vi "Slice Engine.vi"(7 "System Parameters":T1={"Optical Parameters"={"Obj. Focal Length [mm]"=0.0, "Scan Lens EFL[mm]"=0.0, "Tube Lens EFL[mm]"=0.0, "Galvo V Range (+/-)"=0.0, "Galvo Max Half Angle [Deg]"=0.0, "Max Galvo Range[%]"=0.0}, "Vibratome"={"Z Bottom [mm]"=0.0, "Pre Cut Dwell [s]"=0.0, "Blade Frequency [RPM]"=0, "Slice Speed [mm/s]"=0.0, "Post Cut Dwell [s]"=0.0, "Ramp Time [s]"=0.0, "Start X [mm]"=0.0, "Start Y [mm]"=0.0, "Slice Length [mm]"=0.0, "Slice Axis"=enum."X Axis", "Controller VISA Ref"="COM4"}, "Table Stages"={"X Stage"={"Position"=0.0, "Is.Enabled?"=FALSE, "Is.Connected?"=FALSE, "Device SN"="45876425", "AccelerationMaximum"=50.0, "VelocityMaximum"=50.0, "Acceleration"=50.0, "Velocity"=50.0, "waitTimeout (ms)"=500000, "Model"=enum."Thorlabs LTS", "Is.Homed?"=FALSE}, "Y Stage"={"Position"=0.0, "Is.Enabled?"=FALSE, "Is.Connected?"=FALSE, "Device SN"="45995820", "AccelerationMaximum"=50.0, "VelocityMaximum"=50.0, "Acceleration"=50.0, "Velocity"=50.0, "waitTimeout (ms)"=500000, "Model"=enum."Thorlabs LTS", "Is.Homed?"=FALSE}, "Z Stage"={"Position"=0.0, "Is.Enabled?"=FALSE, "Is.Connected?"=FALSE, "Device SN"="49103464", "AccelerationMaximum"=10.0, "VelocityMaximum"=5.0, "Acceleration"=10.0, "Velocity"=5.0, "waitTimeout (ms)"=100000, "Model"=enum."Thorlabs MLJ", "Is.Homed?"=FALSE}}, "Imaging Parameter"={"Raster Scan Direction"=enum."Uni Directional", "Pixel Dwell Time [Clock Cycles]"=0, "Flyback Time [Clock Cycles]"=0, "XY Center [um]"={"X"=1.0, "Y"=1.0}, "Pixel Step Size [um]"=0.0, "XY Image Size"=enum."32 x 32", "Custom"=FALSE, "Custom Size"={"X"=1, "Y"=1}, "Line Averages"=1}, "Galvo HW Parameters"={"Analog Out Channel"="GalvoCtrl/ao0,GalvoCtrl/ao1", "Min Voltage"=-10.0, "Max Voltage"=10.0, "Pixel Clock Source"="/GalvoCtrl/PFI0", "Sample Rate"=1000.0, "Line Clock Out Ch"="GalvoCtrl/port0/line0"}, "Alazar parameters"={"Trigger Settings"={"General Trigger Settings"={"Trigger Operation"=0, "Coupling ID"=2, "Range ID"=2, "Delay"=0, "Timeout Ticks"=0, "Mode"=1, "Parameter"=1}, "Trigger Engine 1"={"Trigger Engine"=0, "Source"=2, "Slope"=1, "Level"=140}, "Trigger Engine 2"={"Trigger Engine"=1000, "Source"=2048, "Slope"=2048, "Level"=140}}, "Capture Clock"={"Sample Rate"=100, "Decimation"=0, "Source"=2, "Edge"=0}, "Device ID"={"System ID"=1, "Board ID"=1}, "Ch A Input Control"={"Channel"=1, "Coupling"=2, "Range"=10, "Impedance"=2}, "Ch B Input Control"={"Channel"=2, "Coupling"=2, "Range"=10, "Impedance"=2}, "Acq Settings"={"Window Type"=1, "Record Length"=1440, "Footer"=0, "Offset"=0, "Records Per Buffer"=2048, "Samples per record"=2048, "Records Count (Records/Acq)"=2147483647, "Output Format"=10}}, "Mosaic Paramter"={"X Axis"={"Start [mm]"=0.0, "Steps [pts]"=0.0, "End [mm]"=0.0}, "Y Axis"={"Start [mm]"=0.0, "Steps [pts]"=0.0, "End [mm]"=0.0}, "Scan Pattern"=enum."Uni-directional", "Overlap Options"={"Overlap Type"=enum."No Overlap", "Percent Overlap"=0, "Justify"=enum."Start"}}, "Vibratome Axis"={"Start [mm]"=95.8, "thick[um]"=2.1, "#slices"=111}} {"Alazar parameters"."Acq Settings"."Output Format" items=["U16_LOG"=1, "U16_AMP2"=257]; "Alazar parameters"."Acq Settings"."Window Type" items=["DSP_WINDOW_NONE", "DSP_WINDOW_HANNING", "DSP_WINDOW_HAMMING", "DSP_WINDOW_BLACKMAN", "DSP_WINDOW_BLACKMAN_HARRIS", "DSP_WINDOW_BARTLETT"]; "Alazar parameters"."Acq Settings"."Footer" items=["FOOTER_NONE", "FOOTER_NPT"]; "Alazar parameters"."Ch B Input Control"."Channel" items=["A"=1, "B"=2, "C"=4, "D"=8]; "Alazar parameters"."Ch B Input Control"."Coupling" items=["AC"=1, "DC"=2]; "Alazar parameters"."Ch B Input Control"."Range" items=["20 mV"=1, "40 mV"=2, "50 mV"=3, "80 mV"=4, "100 mV"=5, "200 mV"=6, "400 mV"=7, "500 mV"=8, "800 mV"=9, "1 V"=10, "1.25 V"=33, "2 V"=11, "4 V"=12, "5 V"=13, "8 V"=14, "10 V"=15, "20 V"=16]; "Alazar parameters"."Ch B Input Control"."Impedance" items=["1 MOhm"=1, "50 Ohm"=2, ""=0]; "Alazar parameters"."Ch A Input Control"."Channel" items=["A"=1, "B"=2, "C"=4, "D"=8]; "Alazar parameters"."Ch A Input Control"."Coupling" items=["AC"=1, "DC"=2]; "Alazar parameters"."Ch A Input Control"."Range" items=["20 mV"=1, "40 mV"=2, "50 mV"=3, "80 mV"=4, "100 mV"=5, "200 mV"=6, "400 mV"=7, "500 mV"=8, "800 mV"=9, "1 V"=10, "1.25 V"=33, "2 V"=11, "4 V"=12, "5 V"=13, "8 V"=14, "10 V"=15, "20 V"=16]; "Alazar parameters"."Ch A Input Control"."Impedance" items=["1 MOhm"=1, "50 Ohm"=2, ""=0]; "Alazar parameters"."Capture Clock"."Edge" items=["Rising", "Falling"]; "Alazar parameters"."Capture Clock"."Source" items=["Internal"=1, "Fast External"=2, "Medium External"=3, "Slow External"=4, "External AC"=5, "External DC"=6, "External 10MHz"=7]; "Alazar parameters"."Trigger Settings"."General Trigger Settings"."Trigger Operation" items=["J", "K", "J OR K", "J AND K", "J XOR K", "J AND NOT K", "NOT J AND K"]; "Alazar parameters"."Trigger Settings"."General Trigger Settings"."Coupling ID" items=["AC"=1, "DC"=2]; "Alazar parameters"."Trigger Settings"."General Trigger Settings"."Range ID" items=["5 V", "1 V", "TTL"]; "Alazar parameters"."Trigger Settings"."Trigger Engine 1"."Trigger Engine" items=["J", "K"]; "Alazar parameters"."Trigger Settings"."Trigger Engine 1"."Source" items=["A", "B", "External", "Disable", "C", "D"]; "Alazar parameters"."Trigger Settings"."Trigger Engine 1"."Slope" items=["Positive"=1, "Negative"=2]; "Alazar parameters"."Trigger Settings"."Trigger Engine 2"."Trigger Engine" items=["J", "K"]; "Alazar parameters"."Trigger Settings"."Trigger Engine 2"."Source" items=["A", "B", "External", "Disable", "C", "D"]; "Alazar parameters"."Trigger Settings"."Trigger Engine 2"."Slope" items=["Positive"=1, "Negative"=2]; "Imaging Parameter"."Line Averages" min=1 max=30 step=1; "Imaging Parameter"."Flyback Time [Clock Cycles]" max=10 step=1; "Imaging Parameter"."Pixel Step Size [um]" min=0.0 max=10.0 step=0.01; "Imaging Parameter"."Custom Size"."Y" min=1 max=30 step=1; "Imaging Parameter"."Custom Size"."X" min=1 max=30 step=1; "Imaging Parameter"."XY Center [um]"."Y" min=1.0 max=30.0 step=1.0; "Imaging Parameter"."XY Center [um]"."X" min=1.0 max=30.0 step=1.0; "Imaging Parameter"."Pixel Dwell Time [Clock Cycles]" max=10 step=1}, 8 "error in (no error)":errorcluster, 11 "Last Slice?":bool) -> (0 "error out":errorcluster)   [LabVIEW 2018]
uses:
  Controls/System Parameters.ctl
  Controls/Optical Parameters.ctl
  Controls/Vibratome Parameters.ctl
  Controls/Translation Stage Parameters.ctl
  Hardware Mfg/Thorlabs Translation Stages/Controls/Translation Stage Cluster.ctl
  Controls/Translation Stage Types.ctl
  Controls/Imaging Parameters.ctl
  Controls/Scan Direction.ctl
  type defines/Alazar parameters.ctl
  Hardware Mfg/AlazarTech SDK/Controls/General Trigger Settings.ctl
  Hardware Mfg/AlazarTech SDK/Controls/Trigger Engine Controls.ctl
  Hardware Mfg/AlazarTech SDK/Controls/Clock Controls.ctl
  Hardware Mfg/AlazarTech SDK/Controls/Alazar Device ID.ctl
  Hardware Mfg/AlazarTech SDK/Controls/Channel Input Controls.ctl
  Hardware Mfg/AlazarTech SDK/Controls/Alazar Acquisition Settings.ctl
  Controls/Queue Manager Actions.ctl
  Controls/QueueNames.ctl
  Hardware Mfg/Thorlabs Translation Stages/Controls/Motion Translation Module Control.ctl
  Controls/Set Get Controls.ctl
panel:
  # "X"
  # "X"
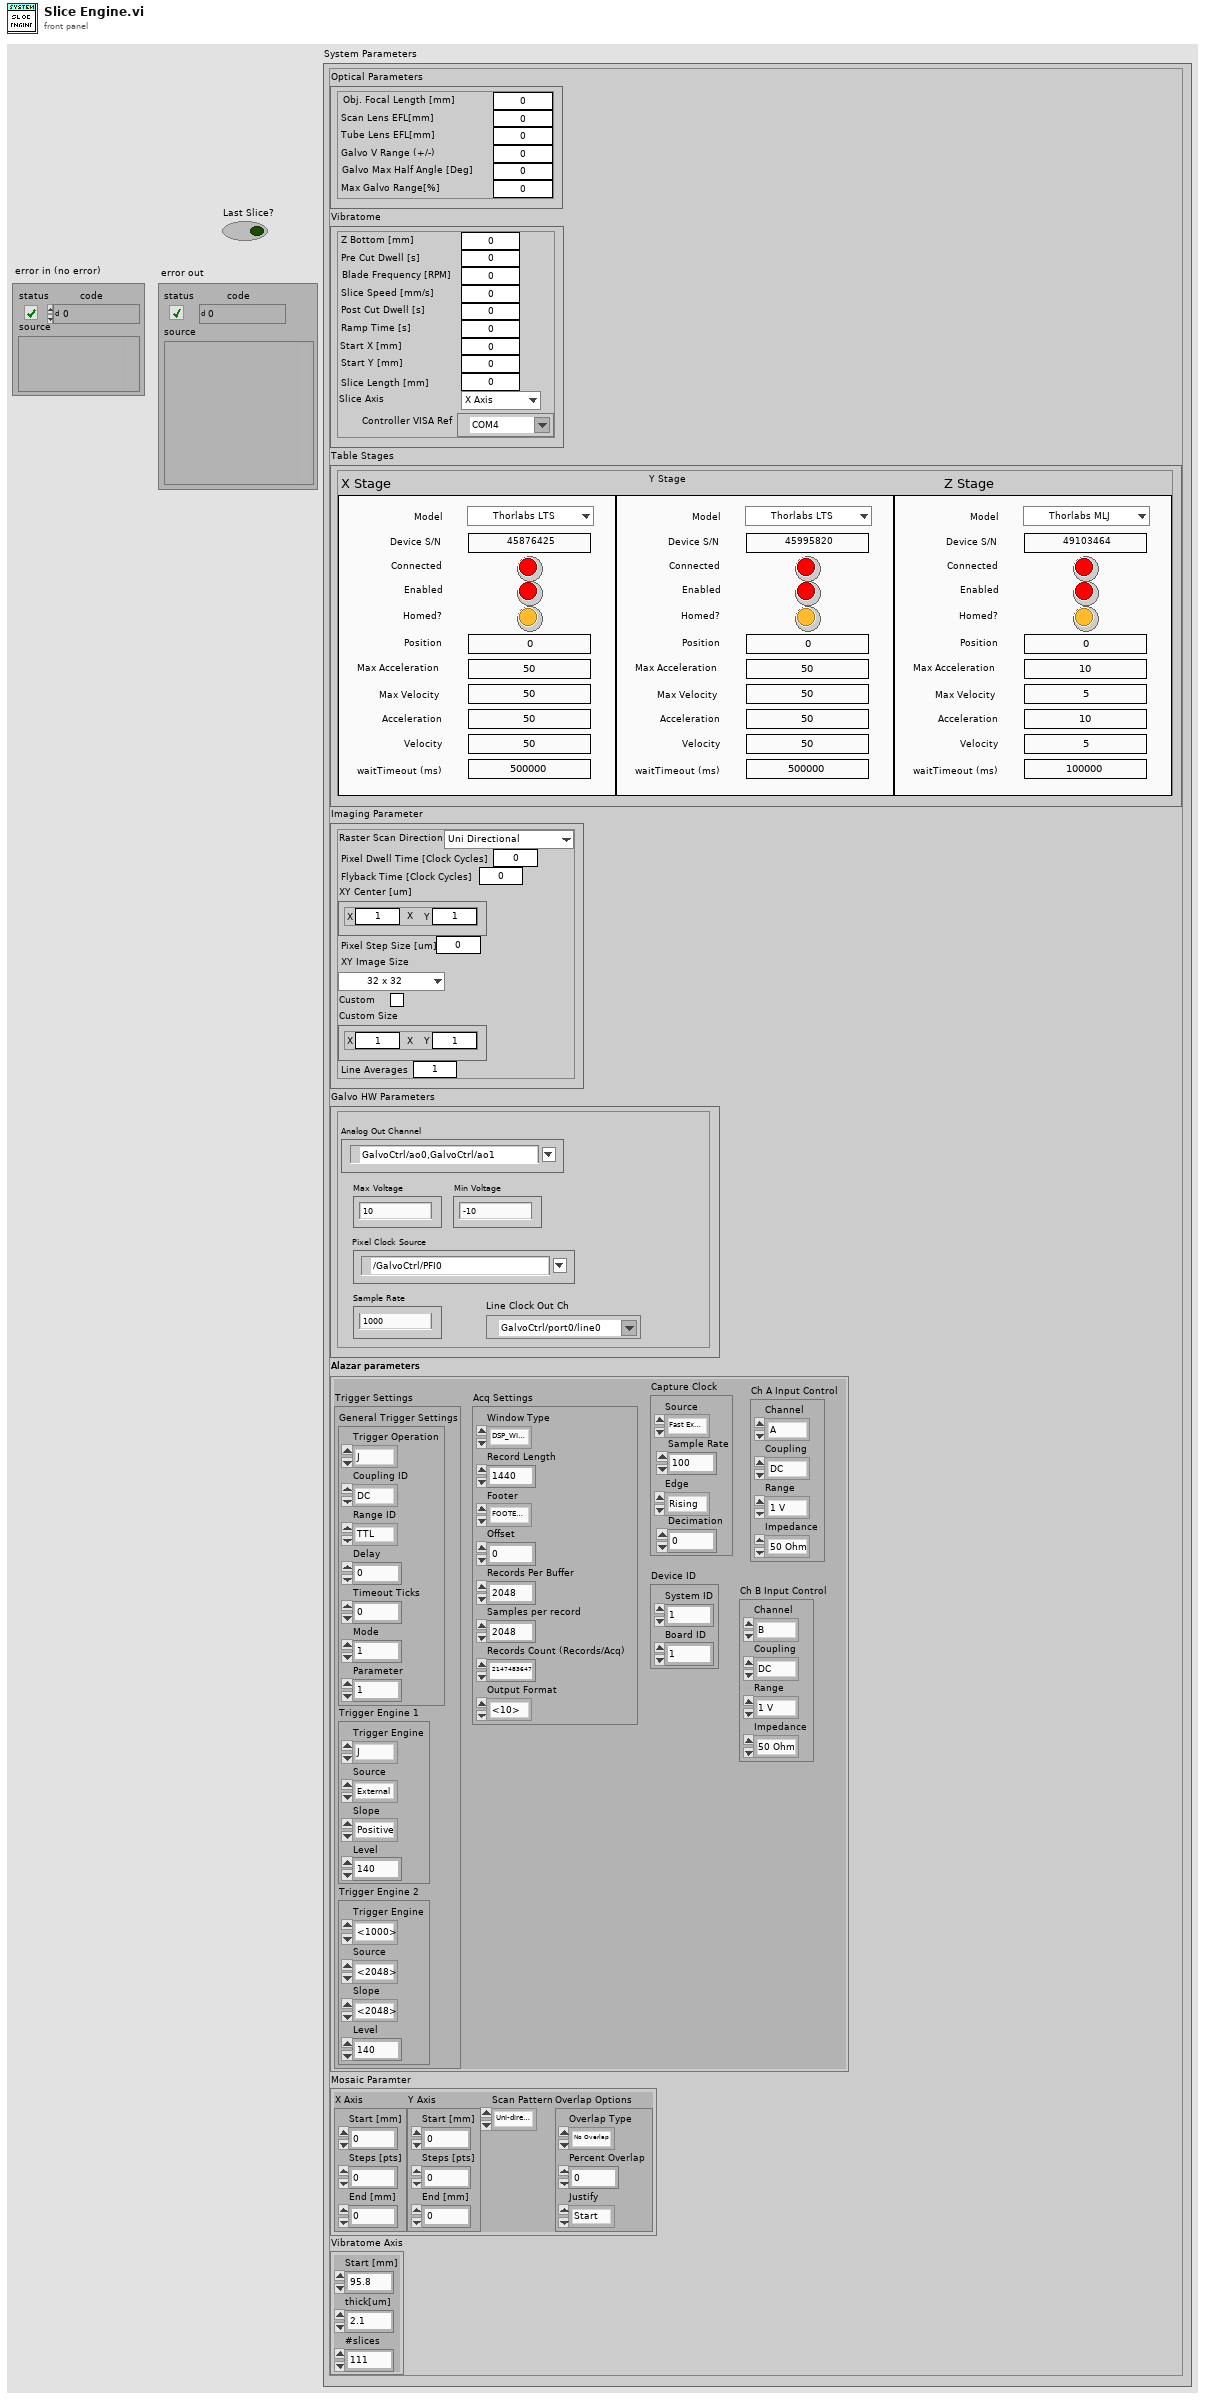
[diagram p1: front panel]
types:
  T1 = typedef "System Parameters.ctl" = cluster{"Optical Parameters":T2, "Vibratome":T3, "Table Stages":T4, "Imaging Parameter":T7, "Galvo HW Parameters":cluster{"Analog Out Channel":tag, "Min Voltage":dbl, "Max Voltage":dbl, "Pixel Clock Source":tag, "Sample Rate":dbl, "Line Clock Out Ch":tag}, "Alazar parameters":T9, "Mosaic Paramter":cluster{"X Axis":cluster{"Start [mm]":dbl, "Steps [pts]":dbl, "End [mm]":dbl}, "Y Axis":cluster{"Start [mm]":dbl, "Steps [pts]":dbl, "End [mm]":dbl}, "Scan Pattern":enum16{"Uni-directional", "Bi-Directional", "Spiral Out", "Spiral In"}, "Overlap Options":cluster{"Overlap Type":enum16{"No Overlap", "X Only", "Y Only", "X and Y"}, "Percent Overlap":u8, "Justify":enum16{"Start", "Center", "End"}}}, "Vibratome Axis":cluster{"Start [mm]":dbl, "thick[um]":dbl, "#slices":u16}}
  T2 = typedef "Optical Parameters.ctl" = cluster{"Obj. Focal Length [mm]":dbl, "Scan Lens EFL[mm]":dbl, "Tube Lens EFL[mm]":dbl, "Galvo V Range (+/-)":dbl, "Galvo Max Half Angle [Deg]":dbl, "Max Galvo Range[%]":dbl}
  T3 = typedef "Vibratome Parameters.ctl" = cluster{"Z Bottom [mm]":dbl, "Pre Cut Dwell [s]":dbl, "Blade Frequency [RPM]":u16, "Slice Speed [mm/s]":dbl, "Post Cut Dwell [s]":dbl, "Ramp Time [s]":dbl, "Start X [mm]":dbl, "Start Y [mm]":dbl, "Slice Length [mm]":dbl, "Slice Axis":enum16{"X Axis", "Y Axis", "Z Axis"}, "Controller VISA Ref":refnum<visa-resource-name>}
  T4 = typedef "Translation Stage Parameters.ctl" = cluster{"X Stage":T5, "Y Stage":T5, "Z Stage":T5}
  T5 = typedef "Translation Stage Cluster.ctl" = cluster{"Position":dbl, "Is.Enabled?":bool, "Is.Connected?":bool, "Device SN":string, "AccelerationMaximum":dbl, "VelocityMaximum":dbl, "Acceleration":dbl, "Velocity":dbl, "waitTimeout (ms)":i32, "Model":T6, "Is.Homed?":bool}
  T6 = typedef "Translation Stage Types.ctl" = enum16{"None", "Thorlabs LTS", "Thorlabs MLJ"}
  T7 = typedef "Imaging Parameters.ctl" = cluster{"Raster Scan Direction":T8, "Pixel Dwell Time [Clock Cycles]":u16, "Flyback Time [Clock Cycles]":u16, "XY Center [um]":cluster{"X":dbl, "Y":dbl}, "Pixel Step Size [um]":dbl, "XY Image Size":enum16{"32 x 32", "64 x 64", "128 x 128", "256 x 256", "512 x 512", "1024 x 1024", "2048 x 2048"}, "Custom":bool, "Custom Size":cluster{"X":u16, "Y":u16}, "Line Averages":u8}
  T8 = typedef "Scan Direction.ctl" = enum16{"Uni Directional", "Bi Directional", "None"}
  T9 = typedef "Alazar parameters.ctl" = cluster{"Trigger Settings":cluster{"General Trigger Settings":T10, "Trigger Engine 1":T11, "Trigger Engine 2":T11}, "Capture Clock":T12, "Device ID":T13, "Ch A Input Control":T14, "Ch B Input Control":T14, "Acq Settings":T15}
  T10 = typedef "General Trigger Settings.ctl" = cluster{"Trigger Operation":u32, "Coupling ID":u32, "Range ID":u32, "Delay":u32, "Timeout Ticks":u32, "Mode":u32, "Parameter":u32}
  T11 = typedef "Trigger Engine Controls.ctl" = cluster{"Trigger Engine":u32, "Source":u32, "Slope":u32, "Level":u32}
  T12 = typedef "Clock Controls.ctl" = cluster{"Sample Rate":u32, "Decimation":u32, "Source":u32, "Edge":u32}
  T13 = typedef "Alazar Device ID.ctl" = cluster{"System ID":u32, "Board ID":u32}
  T14 = typedef "Channel Input Controls.ctl" = cluster{"Channel":u8, "Coupling":u32, "Range":u32, "Impedance":u32}
  T15 = typedef "Alazar Acquisition Settings.ctl" = cluster{"Window Type":u32, "Record Length":u32, "Footer":u32, "Offset":u32, "Records Per Buffer":u32, "Samples per record":u32, "Records Count (Records/Acq)":u32, "Output Format":u32}
  T16 = typedef "QueueNames.ctl" = enum16{"Main GUI", "Main Scan Processor", "Main Processing", "Main Saving", "Main Display", "Main Table Stage GUI", "Main Table Stage Proc.", "Scan Engine", "Vibratome GUI", "Vibratome Processor", "Slice Engine"}
  T17 = typedef "Queue Manager Actions.ctl" = enum16{"Init", "Enqueue", "Enqueue All", "Preview Queue", "Dequeue", "Get Status", "Flush Queue", "Flush All Queues", "Release All Queues", "Release Queue", "Enqueue at Opposite End"}
  T18 = typedef "Set Get Controls.ctl" = enum16{"Set", "Get"}
  T19 = typedef "Motion Translation Module Control.ctl" = enum16{"Init", "Home", "Status", "Velocity/Accel", "Position", "Jog", "Stop", "Uninit", "Enable", "Disable"}
  T20 = enum16{"Set Configuration", "Get Configuration", "Enable Motor", "Disable Motor", "Get Status", "Open Session", "Close Session", "Set Limits", "Get Limits"}
  T21 = cluster{"Source for Velocity":enum16{"Interface", "Voltage (AI)", "PWM (AI)", "Current Target (AI)", "Current Target w/ Preset (AI)"}, "Mode":enum16{"Continuous", "Stepper Motor", "Analog Position Ctrl", "Encoder"}, "Target Velocity [RPM]":i16}
  T22 = typedef "MessagePacket.ctl" = cluster{"Message":string, "Parameter":variant}
  T23 = typedef "Translation Stage Quick Status.ctl" = cluster{"Is.Enabled?":bool, "Is.Connected?":bool, "Is.Homed?":bool}
  T24 = enum16{"Left Button", "Center Button", "Right Button", "Window Close"}
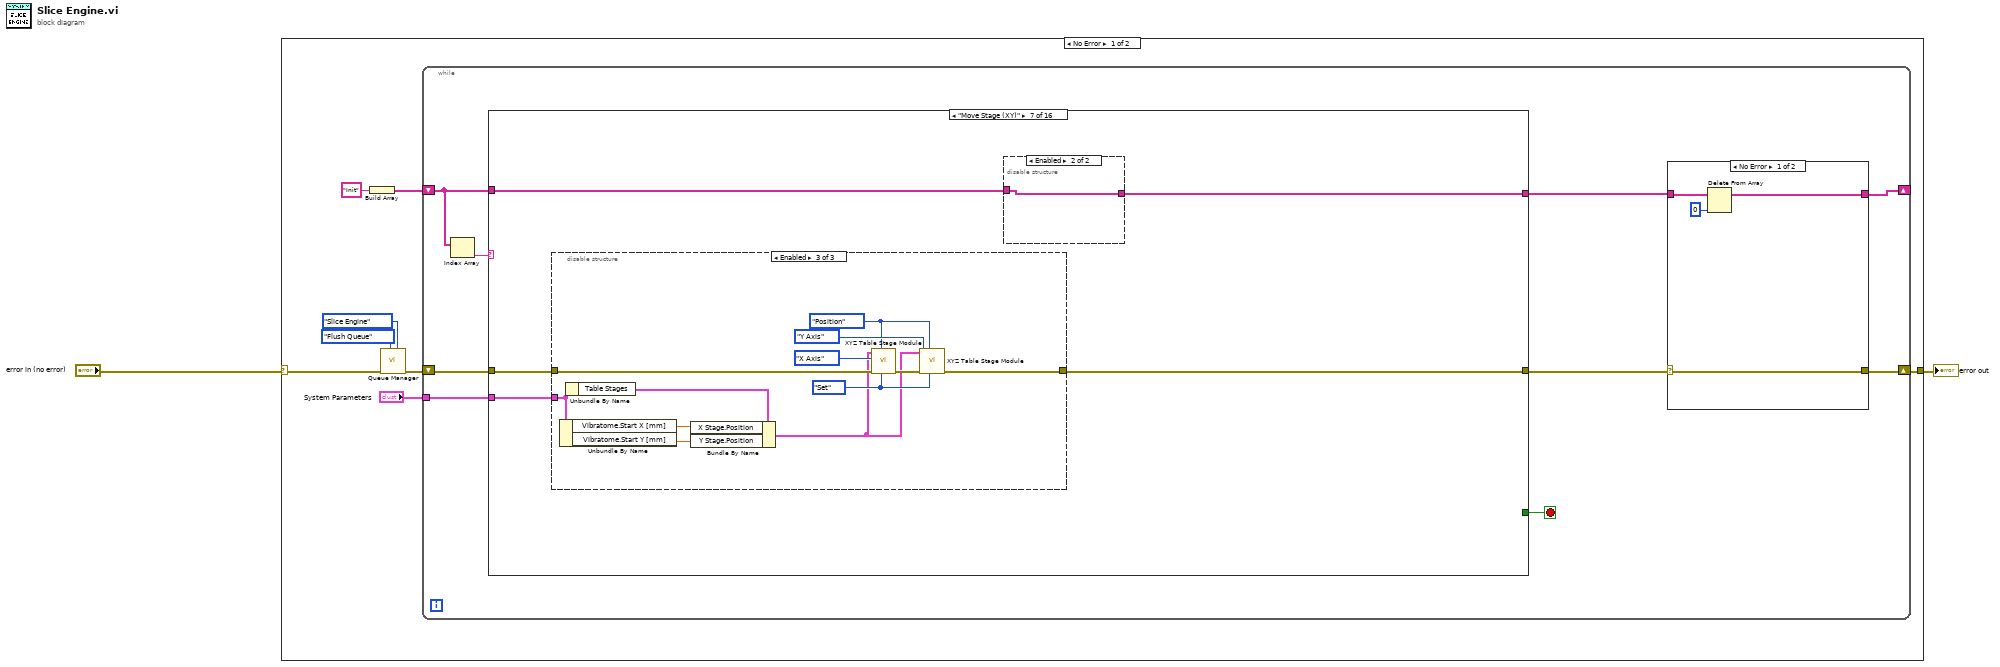
[diagram p0: block diagram]
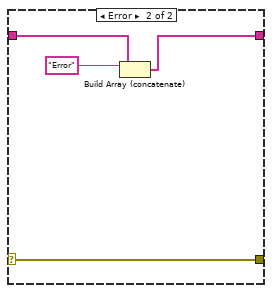
[diagram p2: hidden frame]
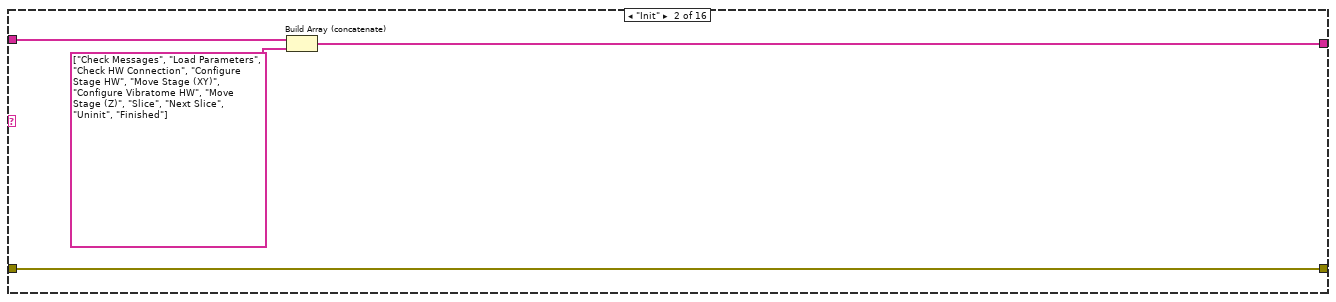
[diagram p4: hidden frame]
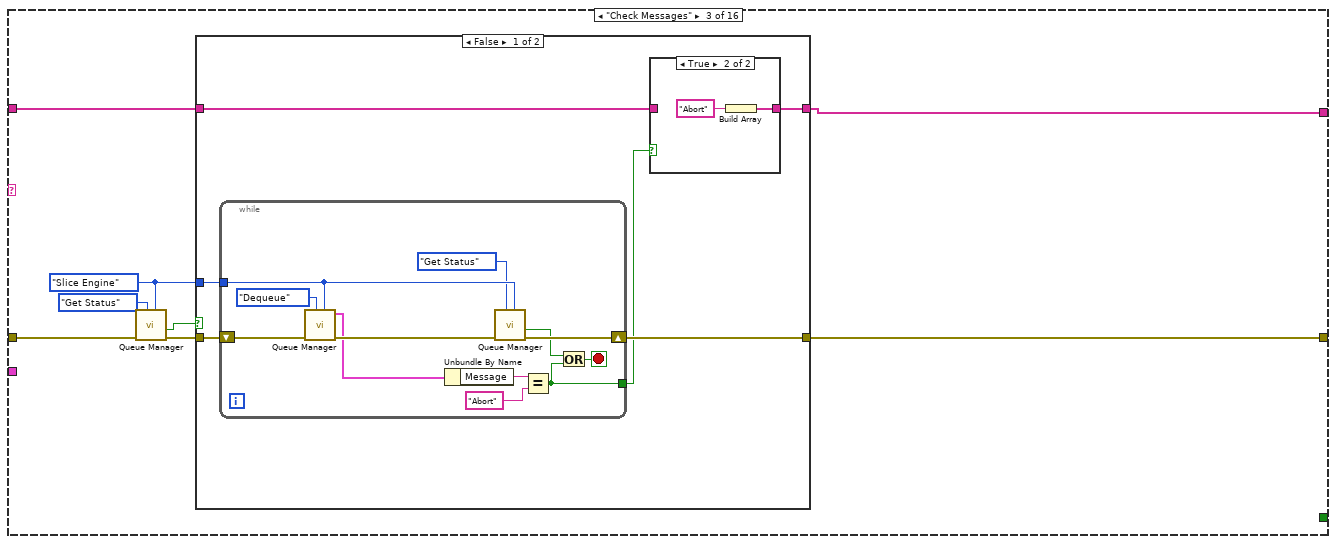
[diagram p5: hidden frame]
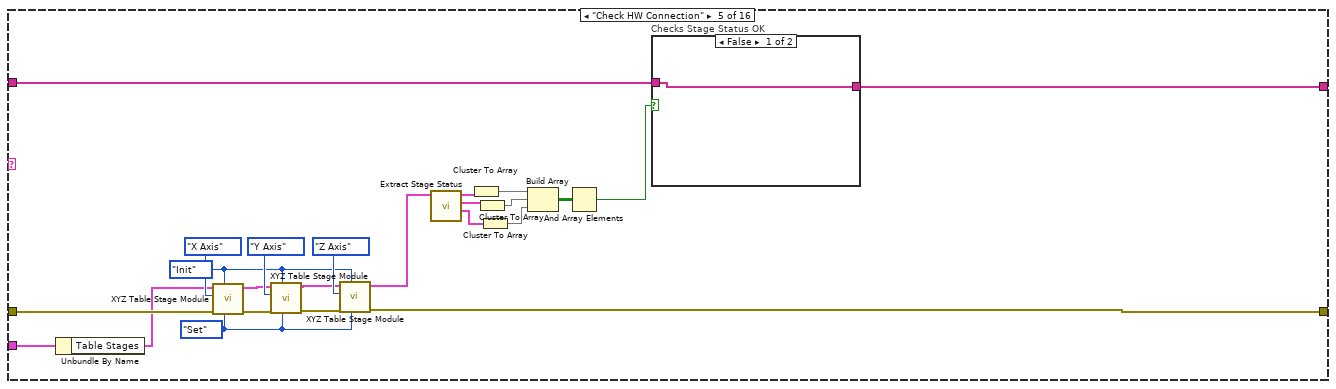
[diagram p9: hidden frame]
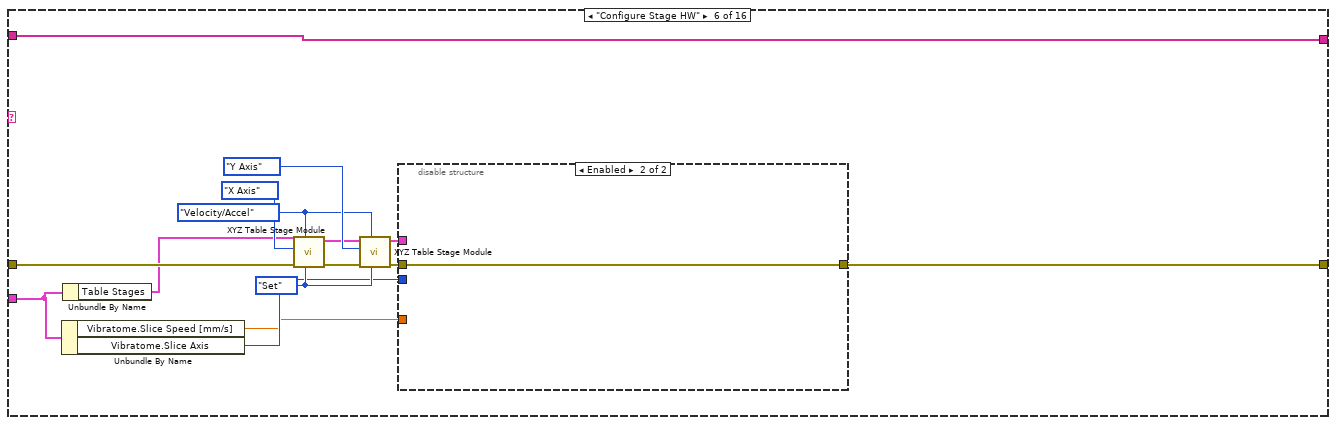
[diagram p11: hidden frame]
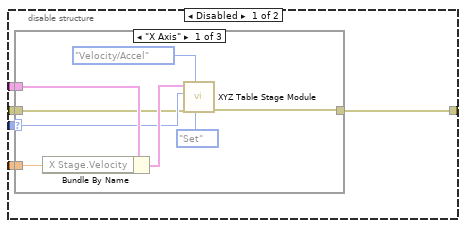
[diagram p12: hidden frame]
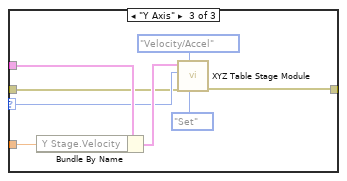
[diagram p14: hidden frame]
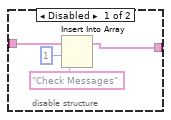
[diagram p15: hidden frame]
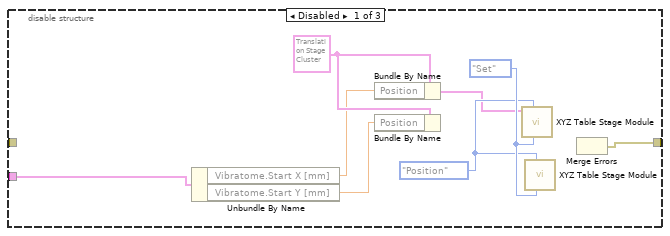
[diagram p16: hidden frame]
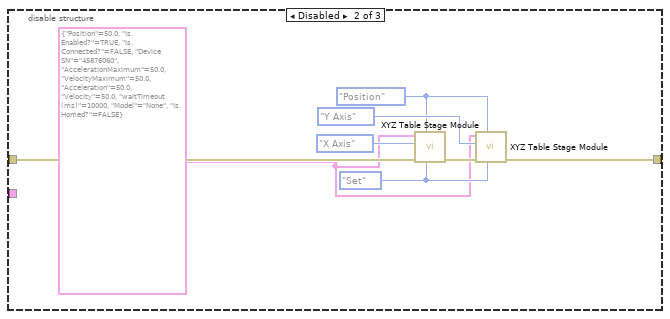
[diagram p17: hidden frame]
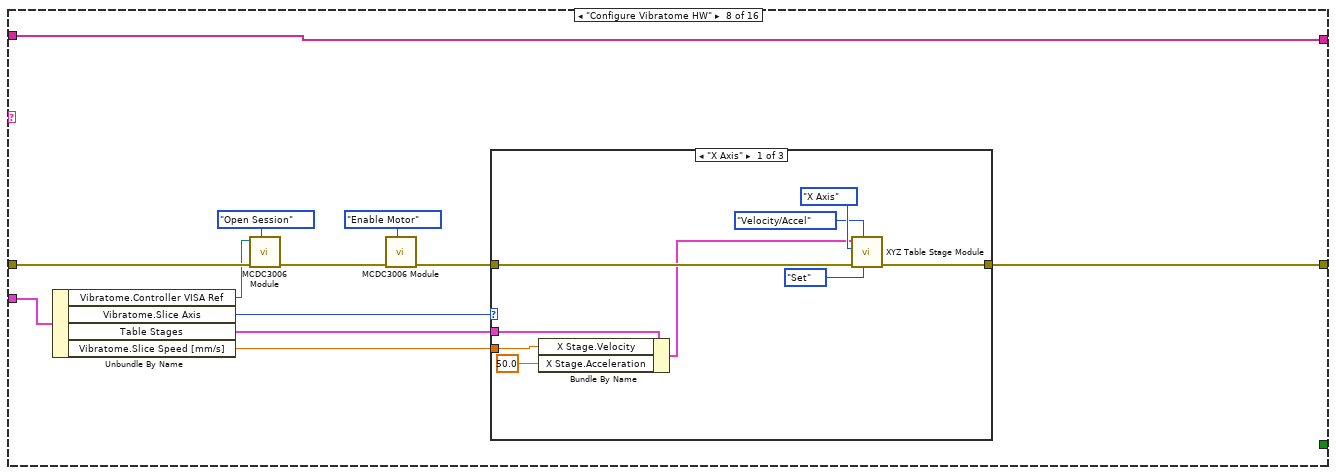
[diagram p18: hidden frame]
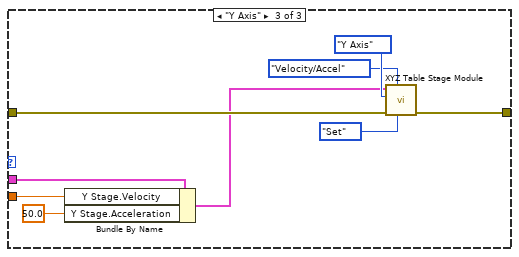
[diagram p20: hidden frame]
diagram:
  n1 = case shown="No Error" "error in (no error)" {
    selector: "error in (no error)" -> [w3 w476]
    tunnel: [w5 w476] -> w1
    frame No Error {
      n2 = Build Array("Init") -> (w6:string[])
      n3 = call "Queue Manager.vi"("Queue Name"=QueueNames."Slice Engine", "Action"=Queue_Manager_Actions."Flush Queue", "Error In"=w3) -> ("Error Out"=w9:errorcluster)  [unwired: 4 in, 4 out]
      n4 = while {
        shift-right: [w13] -> _
        shift-left: w6 -> [w12]
        shift-right: [w15] -> w5
        shift-left: w9 -> [w19]
        tunnel: "System Parameters" -> [w11]
        stop <- w17 stop-if-true
        n5 = Index Array(array=w12) -> (element=w18:string)  [unwired: 1 in]
        n6 = case shown="\"Move Stage (XY)\"" w18 {
          tunnel: w19 -> [w28 w30 w41 w65 w90 w106 w133 w178 w201 w228 w324 w350 w364 w368 w397 w473]
          tunnel: w12 -> [w29 w33 w35 w66 w68 w107 w135 w180 w204 w231 w322 w353 w361 w366 w398 w475]
          tunnel: [w29 w32 w34 w66 w69 w107 w134 w180 w203 w230 w322 w352 w362 w365 w398 w475] -> w14
          tunnel: [_ _ _ _ _ _ _ _ _ _ _ _ _ _ _ TRUE] -> w17
          tunnel: [w28 w30 w36 w65 w88 w93 w132 w172 w202 w229 w323 w350 w364 w369 w395 w472] -> w16
          tunnel: w11 -> [_ _ _ _ w89 w105 w131 w179 w200 w227 w325 _ _ _ w396 _]
          frame "Unknown", Default {
          }
          frame "Init" {
            n7 = Build Array (concatenate)(w33, string[] ["Check Messages", "Load Parameters", "Check HW Connection", "Configure Stage HW", "Move Stage (XY)", "Configure Vibratome HW", "Move Stage (Z)", "Slice", "Next Slice", "Uninit", "Finished"]) -> (w32:string[])
          }
          frame "Check Messages" {
            w37 = QueueNames."Slice Engine" ("Queue Name")
            n8 = call "Queue Manager.vi"("Queue Name"=w37, "Action"=Queue_Manager_Actions."Get Status", "Error In"=w41) -> ("Error Out"=w38:errorcluster, "Empty?"=w39:bool)  [unwired: 4 in, 3 out]
            n9 = case shown="False" w39 {
              tunnel: w38 -> [w47 w63]
              tunnel: w37 -> [w46 _]
              tunnel: [w45 w63] -> w36
              tunnel: w35 -> [w43 w64]
              tunnel: [w42 w64] -> w34
              frame False {
                n10 = while {
                  tunnel: w46 -> [w58]
                  shift-right: [w59] -> w45
                  shift-left: w47 -> [w62]
                  tunnel: [w51] -> w44
                  stop <- w52 stop-if-true
                  n11 = call "Queue Manager.vi"("Queue Name"=w58, "Action"=Queue_Manager_Actions."Dequeue", "Error In"=w62) -> ("Error Out"=w60:errorcluster, "Message Packet [Out]"=w56:T22)  [unwired: 4 in, 3 out]
                  n12 = Unbundle By Name(w56) -> ("Message"=w55:string)
                  n13 = call "Queue Manager.vi"("Queue Name"=w58, "Action"=Queue_Manager_Actions."Get Status", "Error In"=w60) -> ("Error Out"=w59:errorcluster, "Empty?"=w53:bool)  [unwired: 4 in, 3 out]
                  n14 = Equal?(x=w55, y="Abort") -> (x = y?=w51:bool)
                  n15 = Or(x=w53, y=w51) -> (x .or. y?=w52:bool)
                }
                n16 = case shown="True" w44 {
                  tunnel: w43 -> [w48 _]
                  tunnel: [w48 w49] -> w42
                  frame False {
                  }
                  frame True {
                    n17 = Build Array("Abort") -> (w49:string[])
                  }
                }
              }
              frame True {
              }
            }
          }
          frame "Load Parameters" {
          }
          frame "Check HW Connection" {
            w81 = Set_Get_Controls."Set" ("Set/Get")
            w82 = Motion_Translation_Module_Control."Init" ("Action")
            n18 = Unbundle By Name(w89) -> ("Table Stages"=w80:T4)
            n19 = call "XYZ Table Stage Module.vi"("Set/Get"=w81, "Action"=w82, "Error In"=w90, "Axis"=enum16{"X Axis", "Y Axis", "Z Axis"}."X Axis", "Table Stages"=w80) -> ("Error Out"=w87:errorcluster, "Table Stages [out]"=w79:T4)  [unwired: 5 in]
            n20 = call "XYZ Table Stage Module.vi"("Set/Get"=w81, "Action"=w82, "Error In"=w87, "Axis"=enum16{"X Axis", "Y Axis", "Z Axis"}."Y Axis", "Table Stages"=w79) -> ("Error Out"=w86:errorcluster, "Table Stages [out]"=w78:T4)  [unwired: 5 in]
            n21 = call "XYZ Table Stage Module.vi"("Set/Get"=w81, "Action"=w82, "Error In"=w86, "Axis"=enum16{"X Axis", "Y Axis", "Z Axis"}."Z Axis", "Table Stages"=w78) -> ("Error Out"=w88:errorcluster, "Table Stages [out]"=w77:T4)  [unwired: 5 in]
            n22 = call "Extract Stage Status.vi"("Table Stages"=w77) -> ("Z Stage"=w74:T23, "Y Stage"=w75:T23, "X Stage"=w76:T23)  [unwired: 8 in]
            n23 = Cluster To Array(cluster=w76) -> (array=w73:bool[])
            n24 = Cluster To Array(cluster=w75) -> (array=w72:bool[])
            n25 = Cluster To Array(cluster=w74) -> (array=w71:bool[])
            n26 = Build Array(w73, w72, w71) -> (w70:bool[][])
            n27 = And Array Elements(Boolean array=w70) -> (logical AND=w67:bool)
            n28 = case "Checks Stage Status OK" shown="False" w67 {
              tunnel: [w91 w92] -> w69
              tunnel: w68 -> [w91 w92]
              frame False {
              }
              frame True {
              }
            }
          }
          frame "Configure Stage HW" {
            w100 = Set_Get_Controls."Set" ("Set/Get")
            w101 = Motion_Translation_Module_Control."Velocity/Accel" ("Action")
            n29 = Unbundle By Name(w105) -> ("Vibratome.Slice Speed [mm/s]"=w96:dbl, "Vibratome.Slice Axis"=w97:enum16{"X Axis", "Y Axis", "Z Axis"})
            n30 = Unbundle By Name(w105) -> ("Table Stages"=w98:T4)
            n31 = call "XYZ Table Stage Module.vi"("Set/Get"=w100, "Action"=w101, "Error In"=w106, "Axis"=enum16{"X Axis", "Y Axis", "Z Axis"}."X Axis", "Table Stages"=w98) -> ("Error Out"=w104:errorcluster, "Table Stages [out]"=w99:T4)  [unwired: 5 in]
            n32 = call "XYZ Table Stage Module.vi"("Set/Get"=w100, "Action"=w101, "Error In"=w104, "Axis"=enum16{"X Axis", "Y Axis", "Z Axis"}."Y Axis", "Table Stages"=w99) -> ("Error Out"=w94:errorcluster, "Table Stages [out]"=w95:T4)  [unwired: 5 in]
            n33 = disable-structure shown="Enabled" {
              disable-tunnel: w97 -> [w112 _]
              disable-tunnel: w96 -> [w111 _]
              disable-tunnel: w95 -> [w110 _]
              disable-tunnel: w94 -> [w109 w130]
              disable-tunnel: [w108 w130] -> w93
              frame Disabled {
                n34 = case shown="\"X Axis\"" w112 {
                  selector: w112 -> [w117 _ w126]
                  tunnel: w111 -> [w120 _ w129]
                  tunnel: w110 -> [w119 _ w128]
                  tunnel: w109 -> [w116 w121 w125]
                  tunnel: [w115 w121 w124] -> w108
                  frame "X Axis" {
                    n35 = Bundle By Name(cluster=w119, "X Stage.Velocity"=w120) -> (w118:T4)
                    n36 = call "XYZ Table Stage Module.vi"("Set/Get"=Set_Get_Controls."Set", "Action"=Motion_Translation_Module_Control."Velocity/Accel", "Error In"=w116, "Axis"=w117, "Table Stages"=w118) -> ("Error Out"=w115:errorcluster)  [unwired: 5 in, 1 out]
                  }
                  frame "Z Axis" {
                  }
                  frame "Y Axis" {
                    n37 = Bundle By Name(cluster=w128, "Y Stage.Velocity"=w129) -> (w127:T4)
                    n38 = call "XYZ Table Stage Module.vi"("Set/Get"=Set_Get_Controls."Set", "Action"=Motion_Translation_Module_Control."Velocity/Accel", "Error In"=w125, "Axis"=w126, "Table Stages"=w127) -> ("Error Out"=w124:errorcluster)  [unwired: 5 in, 1 out]
                  }
                }
              }
              frame Enabled {
              }
            }
          }
          frame "Move Stage (XY)" {
            n39 = disable-structure shown="Enabled" {
              disable-tunnel: w133 -> [_ w154 w166]
              disable-tunnel: [w148 w155 w167] -> w132
              disable-tunnel: w131 -> [w146 _ w161]
              frame Disabled {
                w147 = T5 {"Position"=0.0, "Is.Enabled?"=TRUE, "Is.Connected?"=FALSE, "Device SN"="45876060", "AccelerationMaximum"=50.0, "VelocityMaximum"=50.0, "Acceleration"=50.0, "Velocity"=50.0, "waitTimeout (ms)"=10000, "Model"=enum."None", "Is.Homed?"=FALSE} ("Cluster In")
                w142 = Motion_Translation_Module_Control."Position" ("Action")
                w143 = Set_Get_Controls."Set" ("Set/Get")
                n40 = Unbundle By Name(w146) -> ("Vibratome.Start X [mm]"=w145:dbl, "Vibratome.Start Y [mm]"=w144:dbl)
                n41 = Bundle By Name(cluster=w147, "Position"=w145) -> (w141:T5)
                n42 = Bundle By Name(cluster=w147, "Position"=w144) -> ()  [unwired: 1 out]
                n43 = call "XYZ Table Stage Module.vi"("Set/Get"=w143, "Action"=w142, "Table Stages"=w141) -> ()  [unwired: 7 in, 2 out]
                n44 = call "XYZ Table Stage Module.vi"("Set/Get"=w143, "Action"=w142) -> ()  [unwired: 8 in, 2 out]
                n45 = Merge Errors() -> (w148:errorcluster)  [unwired: 2 in]
              }
              frame Disabled {
                w150 = Set_Get_Controls."Set" ("Set/Get")
                w151 = Motion_Translation_Module_Control."Position" ("Action")
                w149 = T5 {"Position"=50.0, "Is.Enabled?"=TRUE, "Is.Connected?"=FALSE, "Device SN"="45876060", "AccelerationMaximum"=50.0, "VelocityMaximum"=50.0, "Acceleration"=50.0, "Velocity"=50.0, "waitTimeout (ms)"=10000, "Model"=enum."None", "Is.Homed?"=FALSE} ("Cluster In")
                n46 = call "XYZ Table Stage Module.vi"("Set/Get"=w150, "Action"=w151, "Error In"=w154, "Axis"=enum16{"X Axis", "Y Axis", "Z Axis"}."X Axis", "Table Stages"=w149) -> ("Error Out"=w156:errorcluster)  [unwired: 5 in, 1 out]
                n47 = call "XYZ Table Stage Module.vi"("Set/Get"=w150, "Action"=w151, "Error In"=w156, "Axis"=enum16{"X Axis", "Y Axis", "Z Axis"}."Y Axis", "Table Stages"=w149) -> ("Error Out"=w155:errorcluster)  [unwired: 5 in, 1 out]
              }
              frame Enabled {
                w162 = Set_Get_Controls."Set" ("Set/Get")
                w163 = Motion_Translation_Module_Control."Position" ("Action")
                n48 = Unbundle By Name(w161) -> ("Vibratome.Start X [mm]"=w159:dbl, "Vibratome.Start Y [mm]"=w158:dbl)
                n49 = Unbundle By Name(w161) -> ("Table Stages"=w160:T4)
                n50 = Bundle By Name(cluster=w160, "X Stage.Position"=w159, "Y Stage.Position"=w158) -> (w157:T4)
                n51 = call "XYZ Table Stage Module.vi"("Set/Get"=w162, "Action"=w163, "Error In"=w166, "Axis"=enum16{"X Axis", "Y Axis", "Z Axis"}."X Axis", "Table Stages"=w157) -> ("Error Out"=w168:errorcluster)  [unwired: 5 in, 1 out]
                n52 = call "XYZ Table Stage Module.vi"("Set/Get"=w162, "Action"=w163, "Error In"=w168, "Axis"=enum16{"X Axis", "Y Axis", "Z Axis"}."Y Axis", "Table Stages"=w157) -> ("Error Out"=w167:errorcluster)  [unwired: 5 in, 1 out]
              }
            }
            n53 = disable-structure shown="Enabled" {
              disable-tunnel: w135 -> [w139 w140]
              disable-tunnel: [w138 w140] -> w134
              frame Disabled {
                n54 = Insert Into Array(array=w139, index=1, new element="Check Messages" ("new element/subarray")) -> (w138:string[])
              }
              frame Enabled {
              }
            }
          }
          frame "Configure Vibratome HW" {
            n55 = Unbundle By Name(w179) -> ("Vibratome.Controller VISA Ref"=w176:refnum<visa-resource-name>, "Vibratome.Slice Axis"=w171:enum16{"X Axis", "Y Axis", "Z Axis"}, "Table Stages"=w169:T4, "Vibratome.Slice Speed [mm/s]"=w170:dbl)
            n56 = call "MCDC3006 Module.vi"("Actions"=T20."Open Session", "Error In"=w178, "VISA resource name"=w176) -> ("Error Out"=w174:errorcluster)  [unwired: 4 in, 4 out]
            n57 = call "MCDC3006 Module.vi"("Actions"=T20."Enable Motor", "Error In"=w174) -> ("Error Out"=w173:errorcluster)  [unwired: 5 in, 4 out]
            n58 = case shown="\"X Axis\"" w171 {
              tunnel: [w189 w190 w199] -> w172
              tunnel: w173 -> [w184 w190 w195]
              tunnel: w170 -> [w185 _ w194]
              tunnel: w169 -> [w182 _ w193]
              frame "X Axis" {
                n59 = Bundle By Name(cluster=w182, "X Stage.Velocity"=w185, "X Stage.Acceleration"=50.0 ("Acceleration")) -> (w181:T4)
                n60 = call "XYZ Table Stage Module.vi"("Set/Get"=Set_Get_Controls."Set", "Action"=Motion_Translation_Module_Control."Velocity/Accel", "Error In"=w184, "Axis"=enum16{"X Axis", "Y Axis", "Z Axis"}."X Axis", "Table Stages"=w181) -> ("Error Out"=w189:errorcluster)  [unwired: 5 in, 1 out]
              }
              frame "Z Axis" {
              }
              frame "Y Axis" {
                n61 = Bundle By Name(cluster=w193, "Y Stage.Velocity"=w194, "Y Stage.Acceleration"=50.0 ("Acceleration")) -> (w191:T4)
                n62 = call "XYZ Table Stage Module.vi"("Set/Get"=Set_Get_Controls."Set", "Action"=Motion_Translation_Module_Control."Velocity/Accel", "Error In"=w195, "Axis"=enum16{"X Axis", "Y Axis", "Z Axis"}."Y Axis", "Table Stages"=w191) -> ("Error Out"=w199:errorcluster)  [unwired: 5 in, 1 out]
              }
            }
          }
          frame "Move Stage (Z)" {
            n63 = disable-structure shown="Enabled" {
              disable-tunnel: [w213 w221] -> w202
              disable-tunnel: w201 -> [w212 w221]
              disable-tunnel: w200 -> [w211 _]
              frame Disabled {
                n64 = Unbundle By Name(w211) -> ("Table Stages"=w210:T4)
                n65 = call "XYZ Table Stage Module.vi"("Set/Get"=Set_Get_Controls."Get", "Action"=Motion_Translation_Module_Control."Position", "Error In"=w212, "Axis"=enum16{"X Axis", "Y Axis", "Z Axis"}."Z Axis", "Table Stages"=w210) -> ("Error Out"=w214:errorcluster, "Table Stages [out]"=w209:T4)  [unwired: 5 in]
                n66 = Unbundle By Name(w209) -> ("Z Stage.Position"=w207:dbl)
                n67 = Add(x=w207, y=0.2) -> (x+y=w205:dbl)
                n68 = Bundle By Name(cluster=w209, "Z Stage.Position"=w205) -> (w208:T4)
                n69 = call "XYZ Table Stage Module.vi"("Set/Get"=Set_Get_Controls."Set", "Action"=Motion_Translation_Module_Control."Position", "Error In"=w214, "Axis"=enum16{"X Axis", "Y Axis", "Z Axis"}."Z Axis", "Table Stages"=w208) -> ("Error Out"=w213:errorcluster)  [unwired: 5 in, 1 out]
              }
              frame Enabled {
              }
            }
            n70 = disable-structure shown="Enabled" {
              disable-tunnel: w204 -> [w225 w226]
              disable-tunnel: [w224 w226] -> w203
              frame Disabled {
                n71 = Insert Into Array(array=w225, index=1, new element="Check Messages" ("new element/subarray")) -> (w224:string[])
              }
              frame Enabled {
              }
            }
          }
          frame "Slice" {
            n72 = disable-structure shown="Enabled" {
              disable-tunnel: [w239 w320] -> w229
              disable-tunnel: w228 -> [w238 w321]
              disable-tunnel: w227 -> [w237 w319]
              frame Enabled {
                n73 = Unbundle By Name(w237) -> ("Vibratome.Blade Frequency [RPM]"=w243:u16, "Vibratome.Slice Axis"=w248:enum16{"X Axis", "Y Axis", "Z Axis"}, "Vibratome.Slice Length [mm]"=w247:dbl, "Vibratome.Post Cut Dwell [s]"=w241:dbl, "Vibratome.Pre Cut Dwell [s]"=w240:dbl)
                n74 = Bundle By Name(cluster=T21 {"Source for Velocity"=enum."Interface", "Mode"=enum."Continuous", "Target Velocity [RPM]"=0} ("Configuration [In]"), "Target Velocity [RPM]"=w243) -> (w242:T21)
                n75 = call "MCDC3006 Module.vi"("Actions"=T20."Set Configuration", "Error In"=w238, "Configuration [In]"=w242) -> ("Error Out"=w246:errorcluster)  [unwired: 4 in, 4 out]
                n76 = case shown="\"X Axis\"" w248 {
                  tunnel: w246 -> [w299 w300 w317]
                  tunnel: [w254 w300 w304] -> w239
                  tunnel: w247 -> [w298 _ w311]
                  tunnel: w241 -> [w296 _ w307]
                  tunnel: w240 -> [w293 _ _]
                  tunnel: w237 -> [w274 _ _]
                  frame "X Axis" {
                    n77 = expression code="x*1000"(w293) -> (w292:dbl)
                    n78 = Unbundle By Name(w274) -> ("Table Stages"=w270:T4)
                    n79 = To Unsigned Long Integer(number=w292) -> (unsigned 32bit integer=w291:u32)
                    n80 = call "Inline Wait.vi"("Error In"=w299, "milliseconds to wait"=w291) -> ("Error Out"=w290:errorcluster)  [unwired: 9 in]
                    n81 = call "XYZ Table Stage Module.vi"("Set/Get"=Set_Get_Controls."Get", "Action"=Motion_Translation_Module_Control."Position", "Error In"=w290, "Axis"=enum16{"X Axis", "Y Axis", "Z Axis"}."X Axis", "Table Stages"=w270) -> ("Error Out"=w288:errorcluster, "Table Stages [out]"=w265:T4)  [unwired: 5 in]
                    n82 = expression code="x*1000"(w296) -> (w295:dbl)
                    n83 = Unbundle By Name(w265) -> ("X Stage.Position"=w269:dbl)
                    n84 = To Unsigned Long Integer(number=w295) -> (unsigned 32bit integer=w294:u32)
                    n85 = Add(x=w269, y=w298) -> (x+y=w297:dbl)
                    n86 = Bundle By Name(cluster=w265, "X Stage.Position"=w297) -> (w286:T4)
                    n87 = call "XYZ Table Stage Module.vi"("Set/Get"=Set_Get_Controls."Set", "Action"=Motion_Translation_Module_Control."Position", "Error In"=w288, "Axis"=enum16{"X Axis", "Y Axis", "Z Axis"}."X Axis", "Table Stages"=w286) -> ("Error Out"=w287:errorcluster)  [unwired: 5 in, 1 out]
                    n88 = call "Inline Wait.vi"("Error In"=w287, "milliseconds to wait"=w294) -> ("Error Out"=w284:errorcluster)  [unwired: 9 in]
                    n89 = call "MCDC3006 Module.vi"("Actions"=T20."Disable Motor", "Error In"=w284) -> ("Error Out"=w268:errorcluster)  [unwired: 5 in, 4 out]
                    n90 = call "XYZ Table Stage Module.vi"("Set/Get"=Set_Get_Controls."Get", "Action"=Motion_Translation_Module_Control."Position", "Error In"=w268, "Axis"=enum16{"X Axis", "Y Axis", "Z Axis"}."Z Axis", "Table Stages"=w265) -> ("Error Out"=w267:errorcluster, "Table Stages [out]"=w249:T4)  [unwired: 5 in]
                    n91 = Unbundle By Name(w249) -> ("Z Stage.Position"=w262:dbl)
                    n92 = Subtract(x=w262, y=0.5) -> (x-y=w260:dbl)
                    n93 = Bundle By Name(cluster=w249, "Z Stage.Position"=w260) -> (w259:T4)
                    n94 = call "XYZ Table Stage Module.vi"("Set/Get"=Set_Get_Controls."Set", "Action"=Motion_Translation_Module_Control."Position", "Error In"=w267, "Axis"=enum16{"X Axis", "Y Axis", "Z Axis"}."Z Axis", "Table Stages"=w259) -> ("Error Out"=w255:errorcluster)  [unwired: 5 in, 1 out]
                    n95 = call "XYZ Table Stage Module.vi"("Set/Get"=Set_Get_Controls."Set", "Action"=Motion_Translation_Module_Control."Velocity/Accel", "Error In"=w255, "Axis"=enum16{"X Axis", "Y Axis", "Z Axis"}."X Axis", "Table Stages"=w265) -> ("Error Out"=w275:errorcluster)  [unwired: 5 in, 1 out]
                    n96 = call "XYZ Table Stage Module.vi"("Set/Get"=Set_Get_Controls."Set", "Action"=Motion_Translation_Module_Control."Position", "Error In"=w275, "Axis"=enum16{"X Axis", "Y Axis", "Z Axis"}."X Axis", "Table Stages"=w265) -> ("Error Out"=w253:errorcluster)  [unwired: 5 in, 1 out]
                    n97 = call "XYZ Table Stage Module.vi"("Set/Get"=Set_Get_Controls."Set", "Action"=Motion_Translation_Module_Control."Position", "Error In"=w253, "Axis"=enum16{"X Axis", "Y Axis", "Z Axis"}."Z Axis", "Table Stages"=w249) -> ("Error Out"=w254:errorcluster)  [unwired: 5 in, 1 out]
                  }
                  frame "Z Axis" {
                  }
                  frame "Y Axis" {
                    w301 = Motion_Translation_Module_Control."Position" ("Action")
                    n98 = expression code="x*1000"(w307) -> (w306:dbl)
                    n99 = call "Thorlabs LTS - Y Stage Module.vi"("Set/Get"=Set_Get_Controls."Get", "Error In"=w317, "Action"=w301) -> ("Error Out"=w316:errorcluster, "Cluster Out"=w302:T5)  [unwired: 7 in]
                    n100 = To Unsigned Long Integer(number=w306) -> (unsigned 32bit integer=w305:u32)
                    n101 = Unbundle By Name(w302) -> ("Position"=w312:dbl)
                    n102 = Add(x=w312, y=w311) -> (x+y=w310:dbl)
                    n103 = Bundle By Name(cluster=w302, "Position"=w310) -> (w309:T5)
                    n104 = call "Thorlabs LTS - Y Stage Module.vi"("Set/Get"=Set_Get_Controls."Set", "Error In"=w316, "Action"=w301, "Cluster In"=w309) -> ("Error Out"=w314:errorcluster)  [unwired: 6 in, 1 out]
                    n105 = call "Inline Wait.vi"("Error In"=w314, "milliseconds to wait"=w305) -> ("Error Out"=w308:errorcluster)  [unwired: 9 in]
                    n106 = call "Thorlabs LTS - Y Stage Module.vi"("Set/Get"=Set_Get_Controls."Set", "Error In"=w308, "Action"=w301, "Cluster In"=w302) -> ("Error Out"=w304:errorcluster)  [unwired: 6 in, 1 out]
                  }
                }
              }
              frame Disabled {
                n107 = Unbundle By Name(w319) -> ("Vibratome"=w318:T3)
                n108 = call "Slice Module.vi"("Error In"=w321, "Vibratome"=w318) -> ("Error Out"=w320:errorcluster)  [unwired: 7 in, 2 out]
              }
            }
            n109 = disable-structure shown="Enabled" {
              disable-tunnel: w231 -> [w235 w236]
              disable-tunnel: [w234 w236] -> w230
              frame Disabled {
                n110 = Insert Into Array(array=w235, index=1, new element="Check Messages" ("new element/subarray")) -> (w234:string[])
              }
              frame Enabled {
              }
            }
          }
          frame "set slice speed" {
            n111 = Unbundle By Name(w325) -> ("Vibratome.Slice Axis"=w328:enum16{"X Axis", "Y Axis", "Z Axis"}, "Table Stages"=w326:T4, "Vibratome.Slice Speed [mm/s]"=w327:dbl)
            n112 = call "MCDC3006 Module.vi"("Actions"=T20."Enable Motor", "Error In"=w324) -> ("Error Out"=w329:errorcluster)  [unwired: 5 in, 4 out]
            n113 = case shown="\"X Axis\"" w328 {
              tunnel: [w339 w340 w349] -> w323
              tunnel: w329 -> [w334 w340 w345]
              tunnel: w327 -> [w335 _ w344]
              tunnel: w326 -> [w332 _ w343]
              frame "X Axis" {
                n114 = Bundle By Name(cluster=w332, "X Stage.Velocity"=w335, "X Stage.Acceleration"=50.0 ("Acceleration")) -> (w331:T4)
                n115 = call "XYZ Table Stage Module.vi"("Set/Get"=Set_Get_Controls."Set", "Action"=Motion_Translation_Module_Control."Velocity/Accel", "Error In"=w334, "Axis"=enum16{"X Axis", "Y Axis", "Z Axis"}."X Axis", "Table Stages"=w331) -> ("Error Out"=w339:errorcluster)  [unwired: 5 in, 1 out]
              }
              frame "Z Axis" {
              }
              frame "Y Axis" {
                n116 = Bundle By Name(cluster=w343, "Y Stage.Velocity"=w344, "Y Stage.Acceleration"=50.0 ("Acceleration")) -> (w341:T4)
                n117 = call "XYZ Table Stage Module.vi"("Set/Get"=Set_Get_Controls."Set", "Action"=Motion_Translation_Module_Control."Velocity/Accel", "Error In"=w345, "Axis"=enum16{"X Axis", "Y Axis", "Z Axis"}."Y Axis", "Table Stages"=w341) -> ("Error Out"=w349:errorcluster)  [unwired: 5 in, 1 out]
              }
            }
          }
          frame "Next Slice" {
            n118 = case shown="True" "Last Slice?" {
              tunnel: w353 -> [w357 w358]
              tunnel: [w356 w358] -> w352
              frame False {
                n119 = Insert Into Array(array=w357, index=1, new element=string[] ["Move Stage (Z)", "set slice speed", "Slice", "Next Slice"]) -> (w356:string[])
              }
              frame True {
              }
            }
          }
          frame "Abort" {
            n120 = Insert Into Array(array=w361, index=1, new element #1="Uninit", new element #2="Finished") -> (w362:string[])
          }
          frame "Error" {
            n121 = control-ref of="This VI"() -> (w379:refnum<vi>)
            n122 = property class="VI"(reference=w379) -> ("Name"=w382:string, "Callers"=w384:string[])  [unwired: 1 in, 2 out]
            n123 = Unbundle(w368) -> ("code"=w378:i32, "source"=w377:string)  [unwired: 1 out]
            n124 = Array To Spreadsheet String(delimiter (Tab)=">", array=w384, 3:"%s" ("format string")) -> (spreadsheet string=w383:string)
            n125 = Format Into String(format string="VI Name: %s\nCallers: %s\nError Code: %d\nError Message: %s", initial string="The following error occurred:\n" ("message"), w382, w383, w378, w377) -> (resulting string=w376:string, error out=w370:errorcluster)  [unwired: 1 in]
            n126 = call <vilib>:"Clear Errors.vi"("error in (no error)"=w370) -> ()  [unwired: 5 in, 2 out]
            n127 = call <vilib>:"Three Button Dialog.vi"("Allow user to close window? (TRUE)"=FALSE, "Window Title (\"\")"="Error" ("Window Title (\"\")"), "Right Button Text (\"Cancel\")"="Abort" ("Right Button Text (\"Cancel\")"), "Center Button Text (\"No\")"="Retry" ("Center Button Text (\"No\")"), "Left Button Text (\"Yes\")"="Continue" ("Left Button Text (\"Yes\")"), "message"=w376) -> ("Which Button?"=w367:T24)  [unwired: 5 in]
            n128 = case shown="\"Right Button\"" w367 {
              tunnel: w366 -> [w389 w393 w394]
              tunnel: [w388 w392 w394] -> w365
              frame "Left Button", Default {
                # "Continue"
                n129 = Delete From Array(array=w389, index=0) -> (array with subset deleted=w388:string[])  [unwired: 1 in, 1 out]
              }
              frame "Right Button" {
                # "Abort"
                n130 = Insert Into Array(array=w393, index=1, new element="Abort") -> (w392:string[])
              }
              frame "Center Button" {
                # "Retry"
              }
            }
            n131 = call <vilib>:"Clear Errors.vi"("error in (no error)"=w368) -> ("error out"=w369:errorcluster)  [unwired: 5 in, 1 out]
          }
          frame "Uninit" {
            n132 = disable-structure shown="Enabled" {
              disable-tunnel: w397 -> [w402 w470]
              disable-tunnel: w396 -> [w401 _]
              disable-tunnel: [w400 w463] -> w395
              frame Enabled {
                n133 = for {
                  N: 4 -> [_]
                  tunnel: [w408] -> w403 mode=indexing
                  tunnel: Motion_Translation_Module_Control."Uninit" ("Action") -> [w407]
                  tunnel: w402 -> [w406]
                  tunnel: w401 -> [w405]
                  i -> [w409]
                  n134 = case shown="3" w409 {
                    tunnel: [w415 w429 w443 w452] -> w408
                    tunnel: w406 -> [w414 w428 w442 w457]
                    tunnel: w407 -> [w413 w427 w441 _]
                    tunnel: w405 -> [w412 w426 w440 _]
                    frame 0, Default {
                      # "X Stage"
                      n135 = Unbundle By Name(w412) -> ("Table Stages.X Stage.Model"=w411:T6, "Table Stages.X Stage.Device SN"=w410:string)
                      n136 = case shown="\"Thorlabs LTS\"" w411 {
                        tunnel: [w416 w423] -> w415
                        tunnel: w414 -> [w416 w422]
                        tunnel: w413 -> [_ w421]
                        tunnel: w410 -> [_ w419]
                        frame "None", Default {
                        }
                        frame "Thorlabs LTS" {
                          n137 = Bundle By Name(cluster=T5 {"Position"=0.0, "Is.Enabled?"=TRUE, "Is.Connected?"=FALSE, "Device SN"="45876539", "AccelerationMaximum"=0.0, "VelocityMaximum"=0.0, "Acceleration"=0.0, "Velocity"=0.0, "waitTimeout (ms)"=0, "Model"=enum."Thorlabs LTS", "Is.Homed?"=FALSE} ("Cluster In"), "Device SN"=w419) -> (w418:T5)
                          n138 = call "Thorlabs LTS - X Stage Module.vi"("Set/Get"=Set_Get_Controls."Set", "Error In"=w422, "Action"=w421, "Cluster In"=w418) -> ("Error Out"=w423:errorcluster)  [unwired: 6 in, 1 out]
                        }
                      }
                    }
                    frame 1 {
                      # "Y Stage"
                      n139 = Unbundle By Name(w426) -> ("Table Stages.Y Stage.Model"=w425:T6, "Table Stages.Y Stage.Device SN"=w424:string)
                      n140 = case shown="\"Thorlabs LTS\"" w425 {
                        tunnel: [w430 w437] -> w429
                        tunnel: w428 -> [w430 w436]
                        tunnel: w427 -> [_ w435]
                        tunnel: w424 -> [_ w433]
                        frame "None", Default {
                        }
                        frame "Thorlabs LTS" {
                          n141 = Bundle By Name(cluster=T5 {"Position"=0.0, "Is.Enabled?"=TRUE, "Is.Connected?"=FALSE, "Device SN"="45876539", "AccelerationMaximum"=0.0, "VelocityMaximum"=0.0, "Acceleration"=0.0, "Velocity"=0.0, "waitTimeout (ms)"=0, "Model"=enum."Thorlabs LTS", "Is.Homed?"=FALSE} ("Cluster In"), "Device SN"=w433) -> (w432:T5)
                          n142 = call "Thorlabs LTS - Y Stage Module.vi"("Set/Get"=Set_Get_Controls."Set", "Error In"=w436, "Action"=w435, "Cluster In"=w432) -> ("Error Out"=w437:errorcluster)  [unwired: 6 in, 1 out]
                        }
                      }
                    }
                    frame 2 {
                      # "Z Stage"
                      n143 = Unbundle By Name(w440) -> ("Table Stages.Z Stage.Model"=w439:T6, "Table Stages.Z Stage.Device SN"=w438:string)
                      n144 = case shown="\"Thorlabs MLJ\"" w439 {
                        tunnel: [w444 w451] -> w443
                        tunnel: w442 -> [w444 w450]
                        tunnel: w441 -> [_ w449]
                        tunnel: w438 -> [_ w447]
                        frame "None", Default {
                        }
                        frame "Thorlabs MLJ" {
                          n145 = Bundle By Name(cluster=T5 {"Position"=0.0, "Is.Enabled?"=TRUE, "Is.Connected?"=FALSE, "Device SN"="45876539", "AccelerationMaximum"=0.0, "VelocityMaximum"=0.0, "Acceleration"=0.0, "Velocity"=0.0, "waitTimeout (ms)"=0, "Model"=enum."Thorlabs MLJ", "Is.Homed?"=FALSE} ("Cluster In"), "Device SN"=w447) -> (w446:T5)
                          n146 = call "Thorlabs MLJ - Z Stage Module.vi"("Set/Get"=Set_Get_Controls."Set", "Error In"=w450, "Action"=w449, "Cluster In"=w446) -> ("Error Out"=w451:errorcluster)  [unwired: 6 in, 1 out]
                        }
                      }
                    }
                    frame 3 {
                      # "Vibratome Motor"
                      n147 = call "MCDC3006 Module.vi"("Actions"=T20."Disable Motor", "Error In"=w457) -> ("Error Out"=w455:errorcluster)  [unwired: 5 in, 4 out]
                      n148 = call "MCDC3006 Module.vi"("Actions"=T20."Close Session", "Error In"=w455) -> ("Error Out"=w453:errorcluster)  [unwired: 5 in, 4 out]
                      n149 = call <vilib>:"Clear Errors.vi"("error in (no error)"=w453) -> ("error out"=w452:errorcluster)  [unwired: 5 in, 1 out]
                    }
                  }
                }
                n150 = Merge Errors(w403) -> (w400:errorcluster)
              }
              frame Disabled {
                w458 = Set_Get_Controls."Set" ("Set/Get")
                w462 = Motion_Translation_Module_Control."Uninit" ("Action")
                n151 = call "XYZ Table Stage Module.vi"("Set/Get"=w458, "Action"=w462, "Error In"=w470, "Axis"=enum16{"X Axis", "Y Axis", "Z Axis"}."X Axis") -> ("Error Out"=w469:errorcluster)  [unwired: 6 in, 1 out]
                n152 = call "XYZ Table Stage Module.vi"("Set/Get"=w458, "Action"=w462, "Error In"=w469, "Axis"=enum16{"X Axis", "Y Axis", "Z Axis"}."Y Axis") -> ("Error Out"=w468:errorcluster)  [unwired: 6 in, 1 out]
                n153 = call "XYZ Table Stage Module.vi"("Set/Get"=w458, "Action"=w462, "Error In"=w468, "Axis"=enum16{"X Axis", "Y Axis", "Z Axis"}."Z Axis") -> ("Error Out"=w465:errorcluster)  [unwired: 6 in, 1 out]
                n154 = call "MCDC3006 Module.vi"("Actions"=T20."Disable Motor", "Error In"=w465) -> ("Error Out"=w464:errorcluster)  [unwired: 5 in, 4 out]
                n155 = call "MCDC3006 Module.vi"("Actions"=T20."Close Session", "Error In"=w464) -> ("Error Out"=w463:errorcluster)  [unwired: 5 in, 4 out]
              }
            }
          }
          frame "Finished" {
            n156 = call "Inline Wait.vi"("Error In"=w473, "milliseconds to wait"=u32 1000) -> ("Error Out"=w472:errorcluster)  [unwired: 9 in]
          }
        }
        n157 = case shown="No Error" w16 {
          selector: w16 -> [w23 w24]
          tunnel: [w23 w24] -> w15
          tunnel: w14 -> [w22 w27]
          tunnel: [w21 w25] -> w13
          frame No Error {
            n158 = Delete From Array(array=w22, index=0) -> (array with subset deleted=w21:string[])  [unwired: 1 in, 1 out]
          }
          frame Error {
            n159 = Build Array (concatenate)("Error", w27) -> (w25:string[])
          }
        }
      }
    }
    frame Error {
    }
  }
  "error out" <- w1
